vi "Create Channel Buffer.vi"(8 "error in":errorcluster, 10 "Channel":string, 11 "BufferLossless in":refnum<class "Buffer Lossless Base.lvclass">) -> (0 "error out":errorcluster, 3 "BufferLossless out":refnum<class "Buffer Lossless Base.lvclass">)   [LabVIEW 2024, in "Buffer Lossless Base.lvclass"]
uses:
  Buffer Lossless Base.lvclass
  Buffer Lossless Base.lvclass/Buffer Lossless Base.ctl
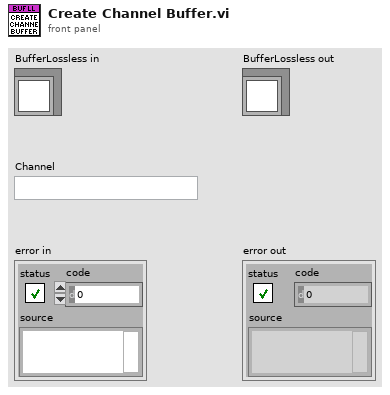
[diagram p1: front panel]
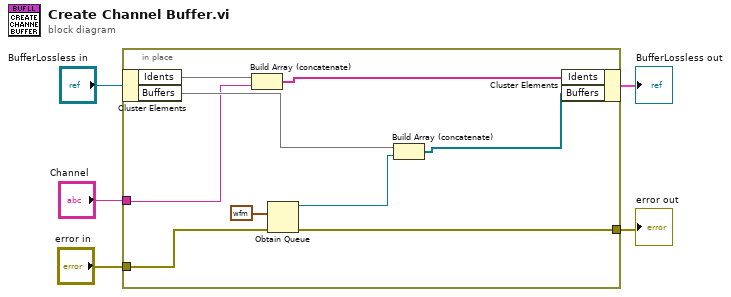
[diagram p0: block diagram]
diagram:
  n1 = in-place {
    in-place-border: [w13] -> w1
    in-place-border: "Channel" -> [w9]
    in-place-border: "error in" -> [w14]
    n2 = in-place-cluster #1("BufferLossless in") -> ("Idents"=w10, "Buffers"=w11)
    n3 = Build Array (concatenate)(w10, w9) -> (w8:string[])
    n4 = Obtain Queue(element data type=waveform(dbl) {"t0"=timestamp(0 s since 1904-01-01), "dt"=1.0, "Y"=[]} ("Waveform"), error in (no error)=w14) -> (queue out=w6:refnum<queue>, error out=w13:errorcluster)  [unwired: 3 in, 1 out]
    n5 = Build Array (concatenate)(w11, w6) -> (w7:refnum<queue>[])
    n6 = in-place-cluster #1("Idents"=w8, "Buffers"=w7) -> (→"BufferLossless out":cluster{})
  }
  "error out" <- w1
